vi "Replace Line.vi"(8 "error in":errorcluster, 9 "New Line":T1, 10 "Line Name":string, 11 "Sequencer Module configuration in":refnum<class "Sequencer Module configuration.lvclass">) -> (0 "error out":errorcluster, 2 "Old Line":T1, 3 "Sequencer Module configuration out":refnum<class "Sequencer Module configuration.lvclass">)   [LabVIEW 2015, in "Sequencer Module configuration.lvclass"]
doc: "Replaces a line identified by name with a new line."
uses:
  Sequencer Module configuration.lvclass
  Line.ctl
  <vilib>/NI/Tag Bus Module Framework/channel/TBM channel.lvclass
  Sequencer Module configuration.lvclass/Sequencer Module configuration.ctl
  <vilib>/NI/Tag Bus Module Framework/module configuration/TBM module configuration.lvclass
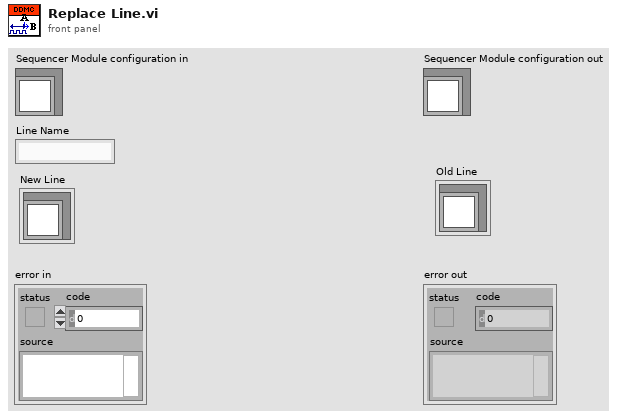
[diagram p1: front panel]
types:
  T1 = typedef "Sequencer Module configuration.lvclass/Line.ctl" = cluster{"channel":refnum<class "TBM channel.lvclass">}
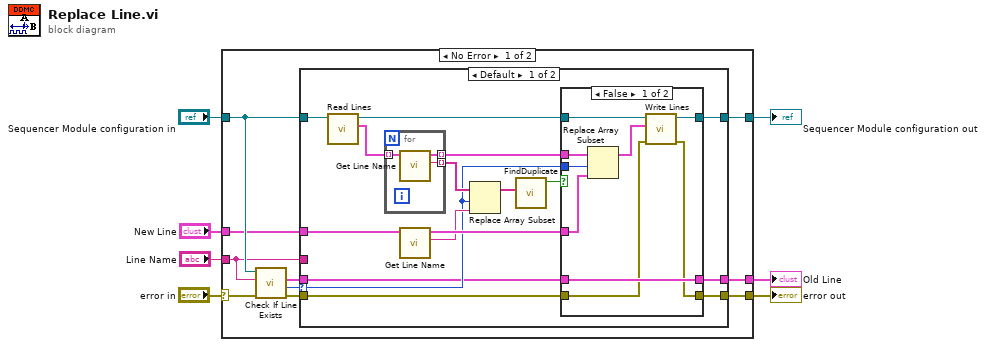
[diagram p0: block diagram]
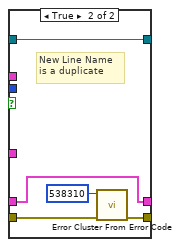
[diagram p2: hidden frame]
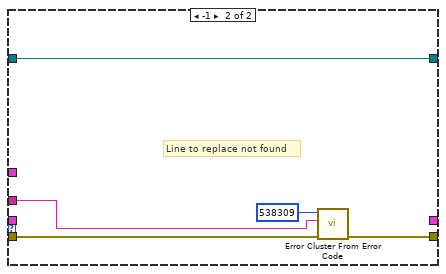
[diagram p3: hidden frame]
diagram:
  n1 = case shown="No Error" "error in" {
    selector: "error in" -> [w11 w57]
    tunnel: [w16 w57] -> w6
    tunnel: [w17 w56] -> w4
    tunnel: "Sequencer Module configuration in" -> [w15 w56]
    tunnel: "Line Name" -> [w14 _]
    tunnel: "New Line" -> [w8 _]
    tunnel: [w12 _] -> w1
    frame No Error {
      n2 = call-dynamic "Check If Line Exists.vi"("error in"=w11, "Name to Locate"=w14, "Sequencer Module configuration in"=w15) -> ("error out"=w10:errorcluster, "Index"=w13:i32, "Line out"=w9:T1)  [unwired: 4 in, 2 out]
      n3 = case shown="Default" w13 {
        selector: w13 -> [w27 _]
        tunnel: w15 -> [w20 w55]
        tunnel: [w33 w55] -> w17
        tunnel: w8 -> [w31 _]
        tunnel: w14 -> [_ w51]
        tunnel: w10 -> [w24 w53]
        tunnel: [w21 w52] -> w16
        tunnel: [w23 _] -> w12
        tunnel: w9 -> [w22 _]
        frame Default {
          n4 = call "Read Lines.vi"("Sequencer Module configuration in"=w20) -> ("Lines"=w18:T1[], "Sequencer Module configuration out"=w19:refnum<class "Sequencer Module configuration.lvclass">)  [unwired: 8 in, 1 out]
          n5 = for {
            tunnel: w18 -> [w50] mode=indexing
            tunnel: [w49] -> w32 mode=indexing
            tunnel: [w48] -> w28 mode=indexing
            n6 = call "Get Line Name.vi"("Line in"=w50) -> ("Name"=w48:string, "Line out"=w49:T1)  [unwired: 8 in, 1 out]
          }
          n7 = call "Get Line Name.vi"("Line in"=w31) -> ("Name"=w29:string, "Line out"=w30:T1)  [unwired: 8 in, 1 out]
          n8 = Replace Array Subset(array=w28, new element=w29, index=w27) -> (w26:string[])
          n9 = call <vilib>:"FindDuplicate.vi"("Array"=w26) -> ("Duplicate"=w25:bool)  [unwired: 8 in, 2 out]
          n10 = case shown="False" w25 {
            tunnel: [w37 w47] -> w33
            tunnel: w19 -> [w38 w47]
            tunnel: w32 -> [w42 _]
            tunnel: w30 -> [w41 _]
            tunnel: w27 -> [w40 _]
            tunnel: w24 -> [w35 w44]
            tunnel: [w39 w46] -> w23
            tunnel: w22 -> [w39 w46]
            tunnel: [w34 w43] -> w21
            frame False {
              n11 = Replace Array Subset(array=w42, new element=w41, index=w40) -> (w36:T1[])
              n12 = call "Write Lines.vi"("error in (no error)"=w35, "Lines"=w36, "Sequencer Module configuration in"=w38) -> ("error out"=w34:errorcluster, "Sequencer Module configuration out"=w37:refnum<class "Sequencer Module configuration.lvclass">)  [unwired: 7 in]
            }
            frame True {
              # "New Line Name\nis a duplicate"
              n13 = call <vilib>:"Error Cluster From Error Code.vi"("error in (no error)"=w44, "error code (0)"=538310) -> ("error out"=w43:errorcluster)  [unwired: 7 in]
            }
          }
        }
        frame -1 {
          # "Line to replace not found"
          n14 = call <vilib>:"Error Cluster From Error Code.vi"("error in (no error)"=w53, "error message (\"\")"=w51, "error code (0)"=538309) -> ("error out"=w52:errorcluster)  [unwired: 6 in]
        }
      }
    }
    frame Error {
    }
  }
  "error out" <- w6
  "Sequencer Module configuration out" <- w4
  "Old Line" <- w1
